vi "Agilent SNA Config Test.vi"(4 "error in (no error)":errorcluster, 6 "Configuration":T1={"BusType"=enum."GPIB", "GPIB Bus"=0, "GPIB Address"=16, "Pass Through Address"=19, "IP"=0, "SCIL Address"=16, "COM"=1, "Baud Rate"=enum."9600", "USB Device"=0, "Instrument S\\N"=""} {"USB Device" max=31 step=1}, 7 "Str Refnum":refnum<vi>) -> (0 "error out":errorcluster, 3 "Serial Number":string)   [LabVIEW 2011]
uses:
  SNA Configuration.ctl
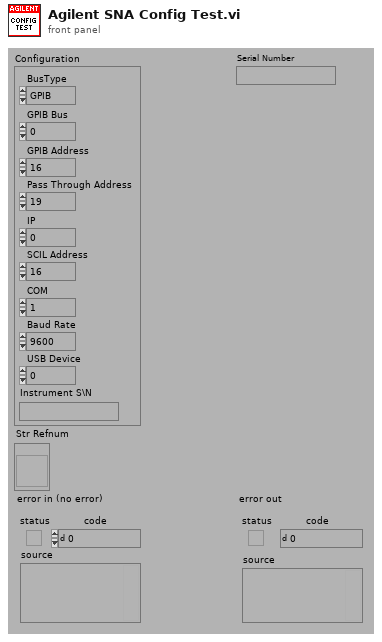
[diagram p1: front panel]
types:
  T1 = typedef "SNA Configuration.ctl" = cluster{"BusType":enum32{"GPIB", "LAN/IP", "Serial", "USB"}, "GPIB Bus":i32, "GPIB Address":i32, "Pass Through Address":i32, "IP":u32, "SCIL Address":i32, "COM":i32, "Baud Rate":enum32{"300", "600", "1200", "2400", "4800", "9600"}, "USB Device":i32, "Instrument S\\N":string}
  T2 = enum32{"300", "600", "1200", "2400", "4800", "9600"}
  T3 = typedef "Agilent SNA VISA.ctl" = cluster{"SNA":refnum<visa-resource-name>, "SNA Pass Through":refnum<visa-resource-name>, "SWP GPIB Address":i32}
  T4 = typedef "Agilent SNA Instrument Info.ctl" = cluster{"SNA":cluster{"Model":string, "Serial":string, "Firmware":string, "Learn String":string}, "SWP":cluster{"Model":string, "Serial":string, "Firmware":string, "Learn String":string}}
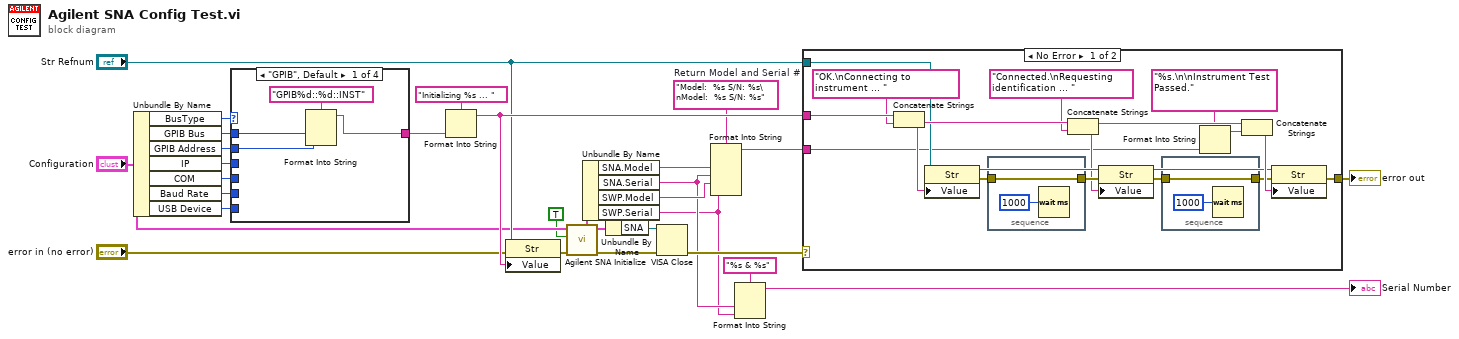
[diagram p0: block diagram]
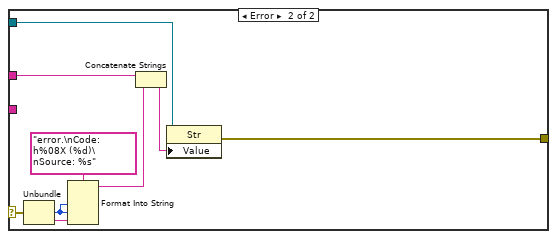
[diagram p2: hidden frame]
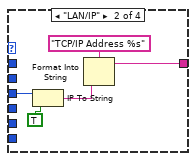
[diagram p3: hidden frame]
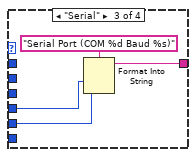
[diagram p4: hidden frame]
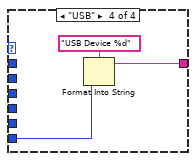
[diagram p5: hidden frame]
diagram:
  w16 = "Model:  %s S/N: %s\nModel:  %s S/N: %s"  # Return Model and Serial #
  n1 = Unbundle By Name("Configuration") -> ("BusType"=w28:enum32{"GPIB", "LAN/IP", "Serial", "USB"}, "GPIB Bus"=w27:i32, "GPIB Address"=w26:i32, "IP"=w25:u32, "COM"=w24:i32, "Baud Rate"=w10:T2, "USB Device"=w9:i32)
  n2 = case shown="\"GPIB\", Default" w28 {
    tunnel: w27 -> [w32 _ _ _]
    tunnel: w26 -> [w31 _ _ _]
    tunnel: w25 -> [_ w37 _ _]
    tunnel: w24 -> [_ _ w41 _]
    tunnel: [w30 w34 w40 w44] -> w23
    tunnel: w10 -> [_ _ w39 _]
    tunnel: w9 -> [_ _ _ w43]
    frame "GPIB", Default {
      n3 = Format Into String(format string="GPIB%d::%d::INST", w32, w31) -> (resulting string=w30:string)  [unwired: 2 in, 1 out]
    }
    frame "LAN/IP" {
      n4 = IP To String(1:TRUE, 2:w37) -> (0:w36:string)
      n5 = Format Into String(format string="TCP/IP Address %s", w36) -> (resulting string=w34:string)  [unwired: 2 in, 1 out]
    }
    frame "Serial" {
      n6 = Format Into String(format string="Serial Port (COM %d Baud %s)", w41, w39) -> (resulting string=w40:string)  [unwired: 2 in, 1 out]
    }
    frame "USB" {
      n7 = Format Into String(format string="USB Device %d", w43) -> (resulting string=w44:string)  [unwired: 2 in, 1 out]
    }
  }
  n8 = Format Into String(format string="Initializing %s ... ", w23) -> (resulting string=w22:string)  [unwired: 2 in, 1 out]
  n9 = property class="Str"(reference="Str Refnum", error in="error in (no error)", "Value"=w22) -> (error out=w18:errorcluster)  [unwired: 1 out]
  n10 = call "Agilent SNA Initialize.vi"("error in (no error)"=w18, "Query Instrument? (T)"=TRUE, "Configuration"="Configuration") -> ("error out"=w14:errorcluster, "VISA Resource Name"=w7:T3, "Agilent SNA & SWP"=w12:T4)  [unwired: 6 out]
  n11 = Unbundle By Name(w12) -> ("SNA.Model"=w15:string, "SNA.Serial"=w4:string, "SWP.Model"=w8:string, "SWP.Serial"=w3:string)
  n12 = Unbundle By Name(w7) -> ("SNA"=w6:refnum<visa-resource-name>)
  n13 = VISA Close(VISA resource name=w6, error in (no error)=w14) -> (error out=w13:errorcluster)
  n14 = Format Into String(format string=w16, w15, w4, w8, w3) -> (resulting string=w11:string)  [unwired: 2 in, 1 out]
  n15 = Format Into String(format string="%s & %s", w4, w3) -> (resulting string=→"Serial Number":string)  [unwired: 2 in, 1 out]
  n16 = case shown="No Error" w13 {
    selector: w13 -> [_ w72]
    tunnel: w22 -> [w58 w75]
    tunnel: [w51 w74] -> w21
    tunnel: "Str Refnum" -> [w49 w71]
    tunnel: w11 -> [w46 _]
    frame No Error {
      n17 = Concatenate Strings(w58, "OK.\nConnecting to instrument ... ") -> (w56:string)
      n18 = property class="Str"(reference=w49, "Value"=w56) -> (reference out=w60:refnum<vi>, error out=w62:errorcluster)  [unwired: 1 in]
      n19 = stacked-sequence {
        tunnel: w62 -> [w65]
        tunnel: [w65] -> w61
        frame #0 {
          n20 = Wait (ms)(milliseconds to wait=u32 1000) -> ()  [unwired: 1 out]
        }
      }
      n21 = Concatenate Strings(w56, "Connected.\nRequesting identification ... ") -> (w52:string)
      n22 = property class="Str"(reference=w60, error in=w61, "Value"=w52) -> (reference out=w50:refnum<vi>, error out=w59:errorcluster)
      n23 = stacked-sequence {
        tunnel: w59 -> [w63]
        tunnel: [w63] -> w53
        frame #0 {
          n24 = Wait (ms)(milliseconds to wait=u32 1000) -> ()  [unwired: 1 out]
        }
      }
      n25 = Format Into String(format string="%s.\n\nInstrument Test Passed.", w46) -> (resulting string=w47:string)  [unwired: 2 in, 1 out]
      n26 = Concatenate Strings(w52, w47) -> (w54:string)
      n27 = property class="Str"(reference=w50, error in=w53, "Value"=w54) -> (error out=w51:errorcluster)  [unwired: 1 out]
    }
    frame Error {
      n28 = Unbundle(w72) -> ("code"=w70:i32, "source"=w69:string)  [unwired: 1 out]
      n29 = Format Into String(format string="error.\nCode:  h%08X (%d)\nSource: %s", w70, w70, w69) -> (resulting string=w68:string)  [unwired: 2 in, 1 out]
      n30 = Concatenate Strings(w75, w68) -> (w67:string)
      n31 = property class="Str"(reference=w71, "Value"=w67) -> (error out=w74:errorcluster)  [unwired: 1 in, 1 out]
    }
  }
  "error out" <- w21
